vi "FPGA Interface.vi"(6 "FIFO CLUSTER IN":T1, 8 "FPGA VI Reference Out 2":refnum<k20>, 10 "RT Main Message Handler":refnum<queue>, 11 "Boolean 2":refnum<vi>) -> ()   [LabVIEW 2017]
uses:
  Support/Message Queue/Message Cluster.ctl
  <vilib>/Platform/TimedLoop/XDataNode/timing_clust.ctl
  <vilib>/Platform/TimedLoop/XDataNode/nitl_modes.ctl
  <vilib>/Platform/TimedLoop/XDataNode/wakeup.ctl
  Controls/Manual Control.ctl
  Globals/RT/Global - Valves.vi
  <vilib>/Utility/error.llb/Error Cluster From Error Code.vi
  <vilib>/rvi/errors/niLvFpgaAdjustHostInterfaceError.vi
  <vilib>/platform/TimedLoop/XDataNode/XDataNode.xnode
  <vilib>/rvi/interface/nirviReadWriteControl/nirviReadWriteControl.xnode
  <vilib>/rvi/interface/nirviMethod/nirviMethod.xnode
  <vilib>/FPGAPlugInAG/Dynamic/niLvFpga_ReadFifo_Dynamic.vi
  <vilib>/rvi/errors/niLvFpgaMergeErrorWithErrorCode.vi
  <vilib>/Platform/TimedLoop/XDataNode/XDNodeRunTimeDep.lvlib
  Support/Message Queue/Message Queue.lvlib
  NiFpgaLv.dll
  <vilib>/rvi/interface/Simulation/niFpgaSimulationCallBeginRW.vi
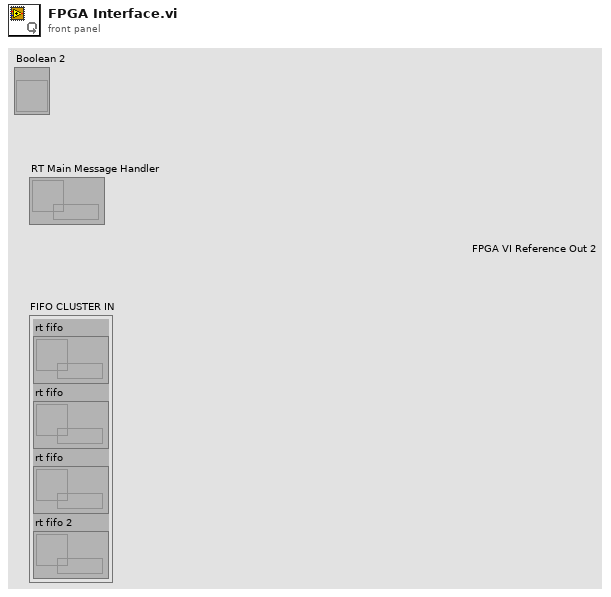
[diagram p1: front panel]
types:
  T1 = cluster{"rt fifo":refnum<k33>, "rt fifo":refnum<k33>, "rt fifo":refnum<k33>, "rt fifo 2":refnum<k33>}
  T2 = enum16{"Manual", "Standby", "Automated Sequence", "Automated Sequence End", "Emergency"}
  T3 = cluster{"Elements Remaining":u32, "Elements Remaining":u32, "Elements Remaining":u32}
  T4 = typedef "XDNodeRunTimeDep.lvlib/timing_clust.ctl" = cluster{"Expected End [f-1]":u64, "Actual End [f-1]":u64, "Finished Late? [f-1]":bool, "Expected End [i-1]":u64, "Actual End [i-1]":u64, "Finished Late? [i-1]":bool, "Expected Start [i]":u64, "Actual Start [i]":u64, "Expected Start [f]":u64, "Actual Start [f]":u64, "Source Name":string, "Structure Name":string, "Period":i64, "Deadline":i64, "Offset":i64, "Start":i64, "Priority":i32, "Timeout":i32, "Mode":T5, "Wakeup Reason":T6, "Error":errorcluster, "Source Type":string, "Secondary Source Type":string, "Global End Time":u64, "Global Start Time":u64, "Frame Duration":u64, "Iteration Duration":u64, "Assigned CPU":i32, "I/O Scan Engine Mode":u32}
  T5 = typedef "XDNodeRunTimeDep.lvlib/nitl_modes.ctl" = enum32{"No Change", "Process missed periods, maintain original phase", "Discard missed periods, maintain original phase", "Process missed periods, ignore original phase", "Discard missed periods, ignore original phase"}
  T6 = typedef "XDNodeRunTimeDep.lvlib/wakeup.ctl" = enum32{"Normal", "Aborted", "Asynchronous wakeup", "Timing source error", "Timed loop error", "Timeout"}
  T7 = cluster{"Unpowered State":u8, "Output Port":u8, "Emergency State":u8, "Blank Button":bool, "Open Time [ms]":fxp<+/-,18,18>, "Close Time [ms]":fxp<+/-,18,18>, "Active":bool}[]
  T8 = typedef "Manual Control.ctl" = cluster{"Actuator Settings":cluster{"Actuator Name":string, "Unpowered State":i16, "Output Port":u32, "Emergency State":i16, "Blank Button":bool, "Open Time [ms]":i16, "Close Time [ms]":i16}[]}
  T9 = cluster{"Actuator Name":string, "Unpowered State":i16, "Output Port":u32, "Emergency State":i16, "Blank Button":bool, "Open Time [ms]":i16, "Close Time [ms]":i16}[]
  T10 = cluster{"Actuator Name":string, "Unpowered State":i16, "Output Port":u32, "Emergency State":i16, "Blank Button":bool, "Open Time [ms]":i16, "Close Time [ms]":i16}
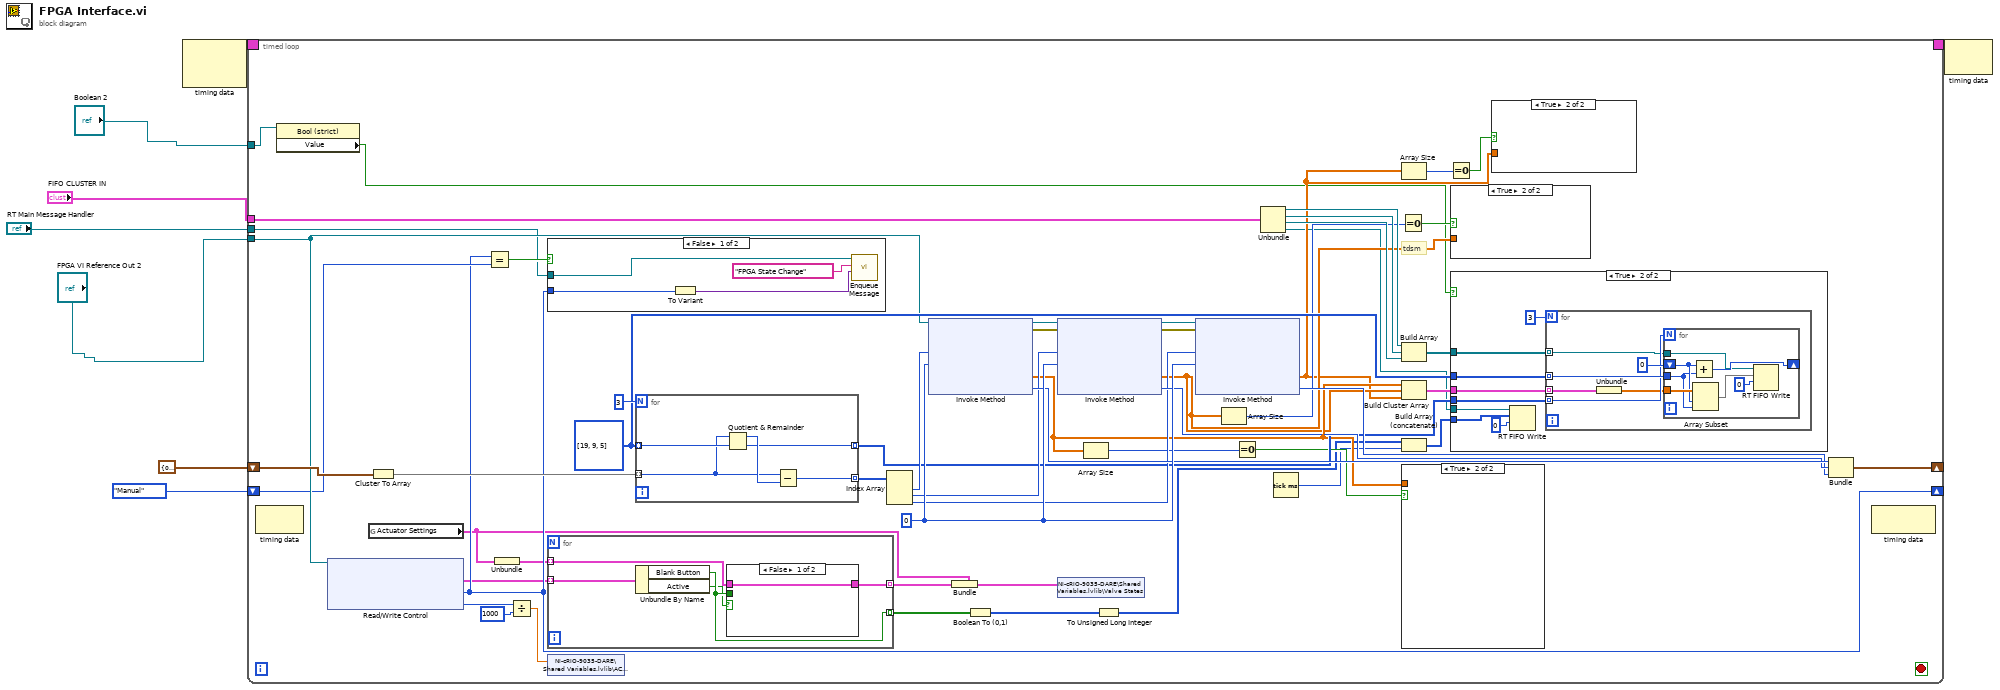
[diagram p0: block diagram]
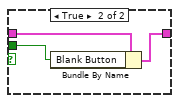
[diagram p2: hidden frame]
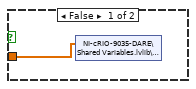
[diagram p5: hidden frame]
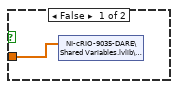
[diagram p6: hidden frame]
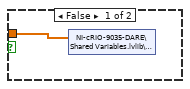
[diagram p7: hidden frame]
diagram:
  n1 = node-c288() -> (w8:T4)  [unwired: 2 in]
  n2 = timed-loop {
    tunnel: "FPGA VI Reference Out 2" -> [w29]
    shift-right: [w54] -> _
    shift-left: T3 {"Elements Remaining"=0, "Elements Remaining"=0, "Elements Remaining"=0} -> [w52]
    tunnel: "FIFO CLUSTER IN" -> [w43]
    timing: w8 -> [_]
    timing-out: [_] -> w7
    shift-right: [w18] -> _
    shift-left: T2."Manual" ("FPGA States") -> [w21]
    tunnel: "RT Main Message Handler" -> [w19]
    tunnel: "Boolean 2" -> [w10]
    stop <- _ stop-if-true
    w45 = i32[] [19, 9, 5]
    w58 = 0 ("Timeout (ms)")
    # "tdsm"
    n3 = node-c288() -> ()  [unwired: 1 in, 1 out]
    n4 = property class="Bool (strict)"(reference=w10) -> ("Value"=w11:bool)  [unwired: 1 in, 2 out]
    n5 = xnode "Read/Write Control"("FPGA VI Reference In"=w29) -> ("Actuator Settings"=w9:T7, "FPGA States"=w18:T2, "Automated Sequence Timer"=w17:i32)  [unwired: 1 in, 2 out]
    n6 = global read "Global - Valves.vi" "Actuator Settings"() -> (w12:T8)
    n7 = Cluster To Array(cluster=w52) -> (array=w51:u32[])
    n8 = Equal?(x=w18, y=w21) -> (x = y?=w20:bool)
    n9 = Unbundle(w12) -> ("Actuator Settings"=w15:T9)
    n10 = Divide(x=w17, y=1000) -> (x/y=w27:dbl)
    n11 = case shown="False" w20 {
      tunnel: w19 -> [w74 _]
      tunnel: w18 -> [w73 _]
      frame False {
        n12 = To Variant(anything=w73) -> (Variant=w72:variant)
        n13 = call "Enqueue Message.vi"("Message Data"=w72, "Message"="FPGA State Change", "Message Queue"=w74) -> ()  [unwired: 7 in, 2 out]
      }
      frame True {
      }
    }
    n14 = for {
      tunnel: w9 -> [w67] mode=indexing
      tunnel: [w65] -> w16 mode=indexing
      tunnel: w15 -> [w66] mode=indexing
      tunnel: [w63] -> w14 mode=indexing
      n15 = Unbundle By Name(w67) -> ("Blank Button"=w65:bool, "Active"=w64:bool)
      n16 = case shown="False" w64 {
        tunnel: w66 -> [w68 w71]
        tunnel: w65 -> [_ w70]
        tunnel: [w68 w69] -> w63
        frame False {
        }
        frame True {
          n17 = Bundle By Name(cluster=w71, "Blank Button"=w70) -> (w69:T10)
        }
      }
    }
    n18 = shared-variable "NI-cRIO-9035-DARE\\Shared Variables.lvlib\\AC Timer"(w27) -> ()  [unwired: 1 in, 1 out]
    n19 = for {
      N: 3 -> [_]
      tunnel: w51 -> [w104] mode=indexing
      tunnel: w45 -> [w106] mode=indexing
      tunnel: [w103] -> w50 mode=indexing
      tunnel: [w102] -> w44 mode=indexing
      n20 = Quotient & Remainder(x=w104, y=w106) -> (x-y*floor(x/y)=w105:u32, floor(x/y)=w102:u32)
      n21 = Subtract(x=w104, y=w105) -> (x-y=w103:u32)
    }
    n22 = Index Array(array=w50) -> (element #1=w49:u32, element #2=w48:u32, element #3=w47:u32)  [unwired: 3 in]
    n23 = xnode "Invoke Method"("FPGA VI Reference In"=w29, "Number of Elements"=w49, "Timeout (ms)"=w58) -> ("FPGA VI Reference Out"=w62:refnum<k20>, "error out"=w61:errorcluster, "Data"=w36:sgl[], "Elements Remaining"=w57:u32)  [unwired: 1 in]
    n24 = Bundle(cluster=w12, "Actuator Settings"=w14) -> (w13:T8)
    n25 = Boolean To (0,1)(Boolean=w16) -> (0, 1=w25:i16[])
    n26 = xnode "Invoke Method"("FPGA VI Reference In"=w62, "error in"=w61, "Number of Elements"=w48, "Timeout (ms)"=w58) -> ("FPGA VI Reference Out"=w60:refnum<k20>, "error out"=w59:errorcluster, "Data"=w31:sgl[], "Elements Remaining"=w56:u32)
    n27 = shared-variable "NI-cRIO-9035-DARE\\Shared Variables.lvlib\\Valve States"(w13) -> ()  [unwired: 1 in, 1 out]
    n28 = Array Size(array=w36) -> (size(s)=w38:i32)
    n29 = To Unsigned Long Integer(number=w25) -> (unsigned 32bit integer=w24:u32[])
    n30 = xnode "Invoke Method"("FPGA VI Reference In"=w60, "error in"=w59, "Number of Elements"=w47, "Timeout (ms)"=w58) -> ("Data"=w30:sgl[], "Elements Remaining"=w55:u32)  [unwired: 2 out]
    n31 = Array Size(array=w31) -> (size(s)=w34:i32)
    n32 = Equal To 0?(x=w38) -> (x = 0?=w37:bool)
    n33 = Unbundle(w43) -> ("rt fifo"=w42:refnum<k33>, "rt fifo"=w41:refnum<k33>, "rt fifo"=w40:refnum<k33>, "rt fifo 2"=w26:refnum<k33>)
    n34 = Tick Count (ms)() -> (millisecond timer value=w22:u32)
    n35 = Equal To 0?(x=w34) -> (x = 0?=w35:bool)
    n36 = Array Size(array=w30) -> (size(s)=w33:i32)
    n37 = Build Array(w42, w41, w40) -> (w39:refnum<k33>[])
    n38 = Build Cluster Array(w36, w31, w30) -> (w46:cluster{"Data":sgl[]}[])
    n39 = Build Array (concatenate)(w24, w22) -> (w23:u32[])
    n40 = case shown="True" w37 {
      tunnel: w36 -> [w101 _]
      frame False {
        n41 = shared-variable "NI-cRIO-9035-DARE\\Shared Variables.lvlib\\TC Data"(w101) -> ()  [unwired: 1 in, 1 out]
      }
      frame True {
      }
    }
    n42 = Equal To 0?(x=w33) -> (x = 0?=w32:bool)
    n43 = case shown="True" w35 {
      tunnel: w31 -> [w100 _]
      frame False {
        n44 = shared-variable "NI-cRIO-9035-DARE\\Shared Variables.lvlib\\PS Data"(w100) -> ()  [unwired: 1 in, 1 out]
      }
      frame True {
      }
    }
    n45 = case shown="True" w11 {
      tunnel: w46 -> [_ w77]
      tunnel: w45 -> [_ w83]
      tunnel: w44 -> [_ w82]
      tunnel: w39 -> [_ w81]
      tunnel: w26 -> [_ w79]
      tunnel: w23 -> [_ w80]
      frame False {
      }
      frame True {
        n46 = RT FIFO Write(0:w79, 1:w80, 2:0 ("timeout in ms (0)")) -> ()  [unwired: 2 in, 4 out]
        n47 = for {
          N: 3 -> [_]
          tunnel: w77 -> [w85] mode=indexing
          tunnel: w83 -> [w89] mode=indexing
          tunnel: w82 -> [w87] mode=indexing
          tunnel: w81 -> [w86] mode=indexing
          n48 = Unbundle(w85) -> ("Data"=w84:sgl[])
          n49 = for {
            N: w87 -> [_]
            tunnel: w84 -> [w96]
            tunnel: w89 -> [w92]
            shift-right: [w91] -> _
            shift-left: 0 ("index") -> [w93]
            tunnel: w86 -> [w90]
            n50 = Add(x=w93, y=w92) -> (x+y=w91:i32)
            n51 = Array Subset(array=w96, index=w93, length=w92) -> (w95:sgl[])
            n52 = RT FIFO Write(0:w90, 1:w95, 2:0 ("timeout in ms (0)")) -> ()  [unwired: 2 in, 4 out]
          }
        }
      }
    }
    n53 = case shown="True" w32 {
      tunnel: w30 -> [w99 _]
      frame False {
        n54 = shared-variable "NI-cRIO-9035-DARE\\Shared Variables.lvlib\\LC Data"(w99) -> ()  [unwired: 1 in, 1 out]
      }
      frame True {
      }
    }
    n55 = Bundle("Elements Remaining"=w57, "Elements Remaining"=w56, "Elements Remaining"=w55) -> (w54:T3)  [unwired: 1 in]
    n56 = node-c288() -> ()  [unwired: 1 in, 1 out]
  }
  n57 = node-c288(w7) -> ()  [unwired: 1 out]
